vi "FPPV.vi"(0 "instrument handle":refnum<k15>="PXI1Slot2 (59)", 1 "Max attempts":dbl=50.0 format="%#_13g", 2 "MLC BLV (V)":dbl=2.0, 5 "Lower resistance (ohm)":dbl, 9 "Upper resistance (ohm)":dbl=6000.0, 11 "error in (no error)":errorcluster, 13 "MLC WLV (V)":dbl=3.0) -> (3 "SL voltage (V)":dbl, 4 "instrument handle out":refnum<k15>="PXI1Slot2 (59)", 6 "final resistance (ohm)":dbl=1580290.44017172 format="%#_6p", 8 "target hit?":bool=TRUE, 10 "final current (A)":dbl=1.265590140368547e-07, 12 "BL voltage (V)":dbl=2.0, 14 "WL voltage (V)":dbl=3.0, 15 "error out":errorcluster)   [LabVIEW 2018]
panel:
  out "attempt number":i32
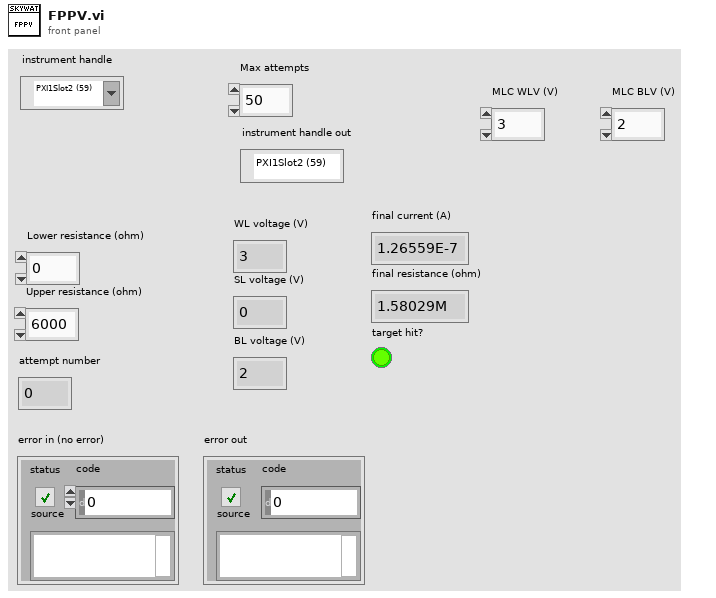
[diagram p1: front panel]
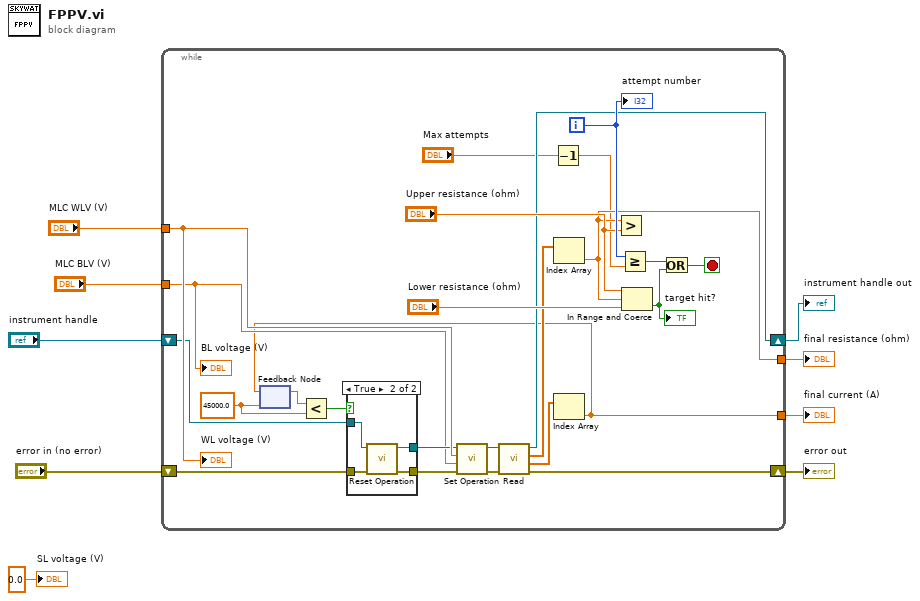
[diagram p0: block diagram]
diagram:
  n1 = while {
    shift-right: [w27] -> w9
    shift-left: "instrument handle" -> [w14]
    shift-right: [w25] -> w8
    shift-left: "error in (no error)" -> [w13]
    tunnel: [w11] -> w4
    tunnel: "MLC WLV (V)" -> [w32]
    tunnel: [w28] -> w3
    tunnel: "MLC BLV (V)" -> [w19]
    i -> [w34]
    stop <- w29 stop-if-true
    w10 = 45000.0 ("y")
    n2 = feedback #1(w10) -> (w12:dbl)
    n3 = Less?(x=w12, y=w10) -> (x < y?=w15:bool)
    n4 = case shown="True" w15 {
      tunnel: [w35 w40] -> w22
      tunnel: [w36 w39] -> w21
      tunnel: w14 -> [w36 w38]
      tunnel: w13 -> [w35 w37]
      frame False {
      }
      frame True {
        n5 = call "Reset Operation.vi"("error in (no error)"=w37, "instrument handle"=w38) -> ("error out"=w40:errorcluster, "instrument handle out"=w39:refnum<k15>)  [unwired: 8 in]
      }
    }
    n6 = call "Set Operation.vi"("error in (no error)"=w22, "BLV"=w19, "WLV"=w32, "instrument handle"=w21) -> ("error out"=w16:errorcluster, "instrument handle out"=w26:refnum<k15>)  [unwired: 6 in]
    n7 = call "Read.vi"("error in (no error)"=w16, "instrument handle"=w26) -> ("error out"=w25:errorcluster, "currents (A)"=w24:dbl[], "resistances (ohm)"=w23:dbl[], "instrument handle out"=w27:refnum<k15>)  [unwired: 6 in]
    n8 = Decrement(x="Max attempts") -> (x-1=w17:dbl)
    n9 = Index Array(array=w23) -> (element=w28:dbl)  [unwired: 1 in]
    n10 = Index Array(array=w24) -> (element=w11:dbl)  [unwired: 1 in]
    n11 = feedback-in #1(w11) -> ()
    n12 = Greater?(x=w28, y="Upper resistance (ohm)") -> ()  [unwired: 1 out]
    n13 = Greater Or Equal?(x=w34, y=w17) -> (x >= y?=w33:bool)
    n14 = In Range and Coerce(upper limit="Upper resistance (ohm)", x=w28, lower limit="Lower resistance (ohm)") -> (In Range?=w20:bool)  [unwired: 1 out]
    "target hit?" <- w20
    n15 = Or(x=w33, y=w20) -> (x .or. y?=w29:bool)
    "attempt number" <- w34
    "WL voltage (V)" <- w32
    "BL voltage (V)" <- w19
  }
  "error out" <- w8
  "instrument handle out" <- w9
  "final current (A)" <- w4
  "final resistance (ohm)" <- w3
  "SL voltage (V)" <- 0.0 ("SL voltage (V)")
